vi "SDF Small Gasifierl HMI - Machine Control Page.vi"(9 "Receiver Process":string="ProcessLoop", 10 "Receiver Host":string) -> ()   [LabVIEW 2013]
uses:
  <vilib>/NI/Current Value Table/DataTypes/String_Read.vi
  <vilib>/NI/Current Value Table/DataTypes/Double_Read.vi
  <vilib>/NI/Current Value Table/Type to Enum.vi
  <vilib>/NI/Current Value Table/DataTypes/String_Type To Enum.vi
  <vilib>/NI/Current Value Table/DataTypes/Double_Type To Enum.vi
  <vilib>/NI/AMC/Create Single Message.vi
  <vilib>/NI/AMC/Update Message Routing Info.vi
  <vilib>/NI/Current Value Table/FGVs/CVT Globals.vi
  <vilib>/NI/Current Value Table/FGVs/Tag Memory.vi
  <vilib>/NI/Current Value Table/Memory Block.vi
  <vilib>/NI/Current Value Table/DataTypes/String_Memory Block.vi
  <vilib>/NI/Current Value Table/DataTypes/Double_Memory Block.vi
  <vilib>/NI/AMC/Send Message.vi
  <vilib>/NI/Current Value Table/Current Value Table.lvlib
  <vilib>/NI/AMC/AMC.lvlib
panel:
  out "Boolean":bool
  out "Value":string
  out "TI-101":dbl
  in  "To Back":bool caption="Caption"
  in  "To CVT Viewer":bool caption="Caption"
  in  "To Alarm Display":bool caption="Caption"
  in  "Stop":bool caption="Caption"
  in  "To Manual Control":bool caption="Caption"
  in  "StartProcess":bool
  out "Page's Title":string="Machine Control"
  # "Home"
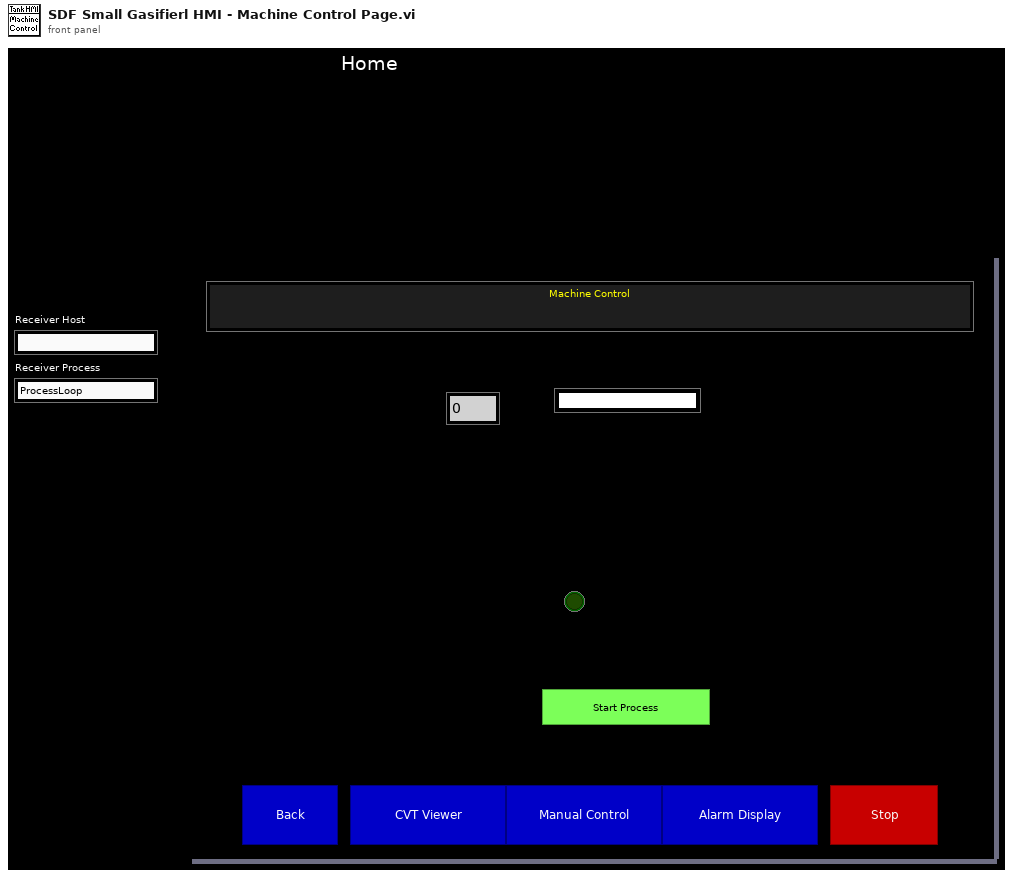
[diagram p1: front panel]
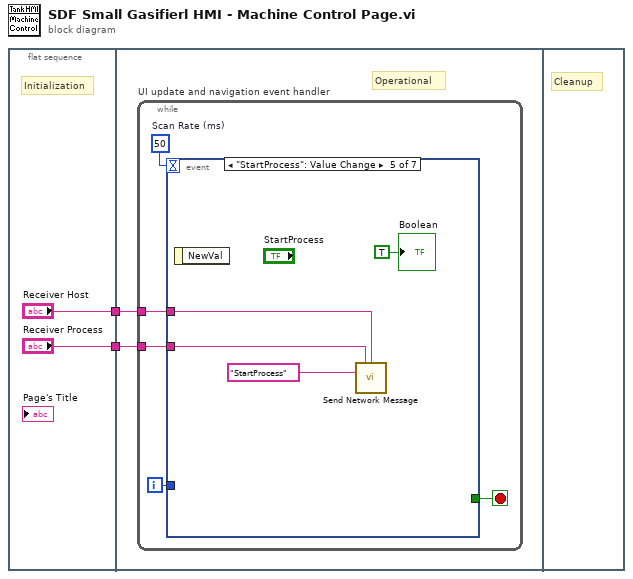
[diagram p0: block diagram]
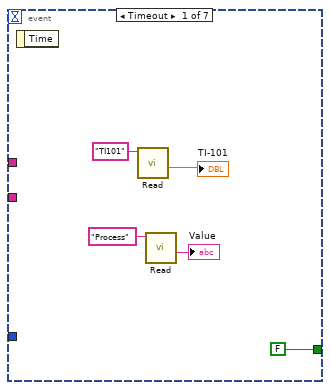
[diagram p2: hidden frame]
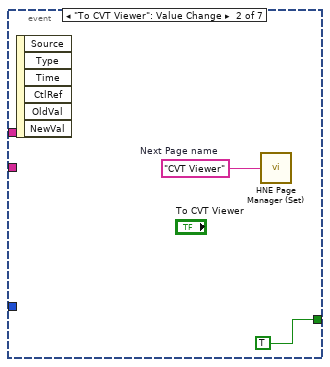
[diagram p3: hidden frame]
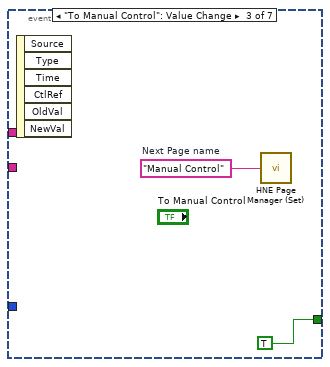
[diagram p4: hidden frame]
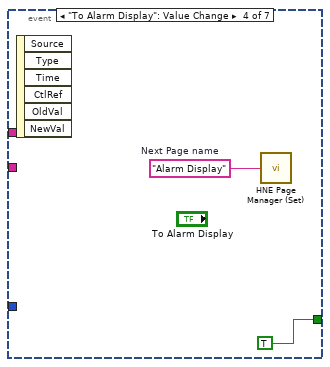
[diagram p5: hidden frame]
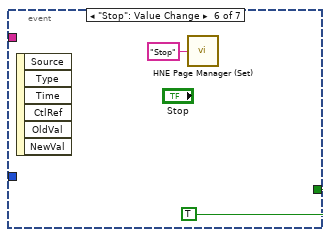
[diagram p6: hidden frame]
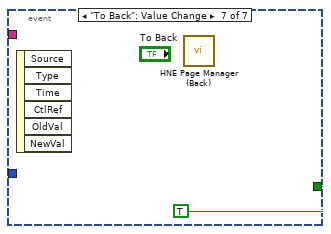
[diagram p7: hidden frame]
diagram:
  n1 = flat-sequence {
    tunnel: ["Receiver Host"] -> w2
    tunnel: ["Receiver Process"] -> w1
    tunnel: w2 -> [w6]
    tunnel: w1 -> [w5]
    frame #0 {
      # "Initialization"
    }
    frame #1 {
      # "Operational"
      n2 = while "UI update and navigation event handler" {
        tunnel: w6 -> [w8]
        tunnel: w5 -> [w7]
        i -> [w10]
        stop <- w11 stop-if-true
        w9 = 50  # Scan Rate (ms)
        n3 = event shown="[4] \"StartProcess\": Value Change" {
          selector: _ -> [_ _ _ _ _ _ _]
          dyn-events: _ -> [_ _ _ _ _ _ _]
          timeout: w9 -> [_ _ _ _ _ _ _]
          tunnel: [FALSE ("Page Name") TRUE ("Page Name") TRUE ("Page Name") TRUE ("Page Name") _ TRUE ("Page Name") TRUE ("Page Name")] -> w11
          tunnel: w10 -> [_ _ _ _ _ _ _]
          tunnel: w8 -> [_ _ _ _ w25 _ _]
          tunnel: w7 -> [_ _ _ _ w24 _ _]
          event Timeout {
            n4 = event-data() -> ()  [unwired: 1 in, 1 out]
            n5 = call-poly <vilib>:"Read.vi"("Tag Name"="TI101") -> ("Value"=→"TI-101":dbl)  [unwired: 9 in, 1 out]
            n6 = call-poly <vilib>:"Read.vi"("Tag Name"="Process") -> ("Value"=→"Value":string)  [unwired: 9 in, 1 out]
          }
          event "To CVT Viewer": Value Change {
            w18 = "CVT Viewer"  # Next Page name
            n7 = event-data() -> ()  [unwired: 1 in, 6 out]
            n8 = call <userlib>:"HNE Page Manager (Set).vi"("Next Page"=w18) -> ()  [unwired: 4 in, 1 out]
          }
          event "To Manual Control": Value Change {
            w20 = "Manual Control"  # Next Page name
            n9 = event-data() -> ()  [unwired: 1 in, 6 out]
            n10 = call <userlib>:"HNE Page Manager (Set).vi"("Next Page"=w20) -> ()  [unwired: 4 in, 1 out]
          }
          event "To Alarm Display": Value Change {
            w22 = "Alarm Display"  # Next Page name
            n11 = event-data() -> ()  [unwired: 1 in, 6 out]
            n12 = call <userlib>:"HNE Page Manager (Set).vi"("Next Page"=w22) -> ()  [unwired: 4 in, 1 out]
          }
          event "StartProcess": Value Change {
            n13 = event-data() -> ()  [unwired: 1 in, 1 out]
            n14 = call <vilib>:"Send Network Message.vi"("receiver process"=w24, "receiver host"=w25, "message name"="StartProcess" ("Tag Name (only if Diff Tag is TRUE)")) -> ()  [unwired: 10 in, 3 out]
            "Boolean" <- TRUE ("Boolean")
          }
          event "Stop": Value Change {
            n15 = event-data() -> ()  [unwired: 1 in, 6 out]
            n16 = call <userlib>:"HNE Page Manager (Set).vi"("Next Page"="Stop") -> ()  [unwired: 4 in, 1 out]
          }
          event "To Back": Value Change {
            n17 = event-data() -> ()  [unwired: 1 in, 6 out]
            n18 = call <userlib>:"HNE Page Manager (Back).vi"() -> ()  [unwired: 5 in, 1 out]
          }
        }
      }
    }
    frame #2 {
      # "Cleanup"
    }
  }
